vi "mode_sensitivity.vi"(0 "reference":refnum<class "OSA.lvclass">, 2 "sensitivity":T1=enum."high", 5 "error in (no error)":errorcluster, 9 "read/write":enum16{"read", "write"}(ring)) -> (14 "duplicate reference":refnum<class "OSA.lvclass">, 16 "sensitivity out":T1=enum."high", 19 "error out":errorcluster)   [LabVIEW 2010, in "OSA.lvclass"]
doc: "Sensitivity affect settable gain range, (sensitivity high: gain range = 0-15, and sens low: 0 - 11), and sampling intervall, (nr of samples per reference laser period, sens high: 32, low: 16). Sensitivity high recommended for low power sources or for high performance wavemeter resolution. The update rate, (interferogram read), is lower in high sensitivity mode."
uses:
  OSA.lvclass
  typeDef/sensitivityMode.ctl
  FTSLib.dll
panel:
  out "status":string
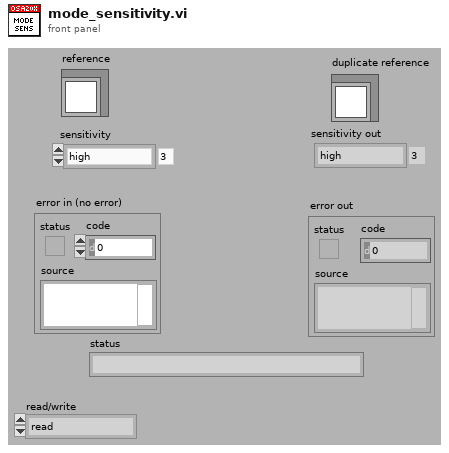
[diagram p1: front panel]
types:
  T1 = typedef "OSA.lvclass/sensitivityMode.ctl" = enum16{"low", "low medium", "high medium", "high"}
  T2 = typedef "OSA.lvclass/ObjectAttributes.ctl" = cluster{"Stop":bool, "dataType":T3, "spectrometerIdx":u16, "buffer size interferogram":i32, "interferogram":cluster{"new":bool, "plot_x_ min":sgl, "plot_x_max":sgl, "plot_y_min":sgl, "plot_y_max":sgl, "Graph Intrfrgrm":T4, "timeStamp":u32, "signal (%)":dbl, "traces":cluster{"idx":u32, "broadBand":bool, "monoChromatic":bool, "peakToPeakSignal":dbl, "peakToPeakPos":dbl}[], "traces idx last":i32}, "spectrum":cluster{"new":bool, "plot_x_min":sgl, "plot_x_max":sgl, "plot_unit_x":T5, "plot_unit_y":T6, "plot_y_min":sgl, "plot_y_max":sgl, "Graph Spectrum":T4, "timeStamp":u32, "X_VAL_OPTIONS":enum16{"MIN_MAX", "ARRAY"}, "traces":cluster{"idx":u32}[], "traces idx last":i32}, "Thorlabs_OSA_64.lvclass:queue_action.ctlqueue ref":refnum<queue>, "action":T7, "plot zoom step":dbl, "buffer semaphore":T8, "acq stopped":bool, "dataType active":T3, "temperature (degr C)":sgl, "pressure (hPa)":sgl, "rel humidity (%)":sgl, "settings":cluster{"resolution":T9, "sensitivity":T1, "Average":bool, "average nr":u32, "apodisation":T10, "acq delay (ms)":u32, "airMesure":T11, "wmtr on":bool, "intfgrm_smooth_width":u16, "intfgrm_smooth_nrOfPasses":u16, "intfgrm_smooth":T12, "phaseCorrection":T13, "zeroFill":u8, "spectr_smooth":T12, "spectr_smooth_width":u16, "spectr_smooth_nrOfPasses":u16, "resolution (/cm)":sgl, "REF wavelength, (nm)":dbl, "gain_idx":u16, "gainAuto":bool, "gain_relative":dbl, "PD sensitivity mode":T14, "PD senseMode implemented":bool, "SensorTemperature implemented":bool, "SensorPressure implemented":bool, "SensorHumidity implemented":bool}, "peaks position":sgl[], "peaks width":sgl[], "peaks height":sgl[], "peaks max nr":u32, "peaks latest nr":i32, "peaks new":bool, "power":dbl, "power new":bool, "path":string, "wavelength (WNr)":dbl, "wavelength new":bool, "buffer size spectrum":i32, "status":string, "VI reference":refnum<vi>, "funcPointer":u64, "libraryPointer":u64, "singleAcquisition":bool, "coherenceLength (cm)":dbl, "coherenceLength new":bool, "spectrometer model":string, "spectrometer serial nr":string, "peaks thld left":sgl[], "peaks thld right":sgl[], "coherenceLength error (cm)":dbl, "ADC bits":u16, "peaks position centroid":sgl[], "peaks height centroid":sgl[], "OSA series":T15, "channel":u16, "channels_nr":i32, "channel stiched":u32, "channelType_spectrum":T16}
  T3 = typedef "OSA.lvclass/acq_dataType.ctl" = enum16{"none", "interferogram", "spectrum"}
  T4 = typedef "OSA.lvclass/graph_intensity.ctl" = refnum<vi>
  T5 = typedef "OSA.lvclass/spectrum_x_unit.ctl" = enum16{"wavenr/cm", "THz", "eV", "nm_air", "nm_vac"}
  T6 = typedef "OSA.lvclass/y_unit.ctl" = enum16{"ADC counts", "dBm pwr absolute", "dBm pwr density", "mW pwr absolute", "mW pwr density"}
  T7 = typedef "OSA.lvclass/queue_action.ctl" = enum16{"none", "stop", "GUI_plotInterferogram", "GUI_plotSpectrum", "GUI_plotInterferogramRescale", "GUI_plotSpectrumRescale", "GUI_plotInterferogramReset", "GUI_plotSpectrumReset", "GUI_plotInterferogramAutoScaleY", "GUI_plotSpectrumAutoScaleY", "GUI_plotInterferogramZoomOut", "GUI_plotSpectrumZoomOut", "GUI_plotInterferogramPane", "GUI_plotSpectrumPane", "GUI_plotInterferogramZoomMouse", "GUI_plotSpectrumZoomMouse", "ENVIRONMENT temperature", "ENVIRONMENT pressure", "MODE_resolution set", "MODE_resolution get", "MODE_sensitivity set", "MODE_sensitivity get", "MODE_PDTemperature set", "MODE_PDTemperature get", "REBOOT/RESET firmware", "ACQASYNC_acquireSingleSpectrum", "ACQASYNC_continuous start", "ACQASYNC_continuous stop\n", "ACQASYNC_get last interferogram", "ACQASYNC_get last spectrum", "ACQASYNC_get last waveNr", "ACQOPT_interferogram smoothing set", "ACQOPT_interferogram smoothing get", "ACQOPT_spectrum smoothing set", "ACQOPT_spectrum smoothing get", "ACQOPT_apodisation type set", "ACQOPT_apodisation type get", "ACQOPT_phase correction type set", "ACQOPT_phase correction type get", "ACQOPT_acqIntervall_set", "ACQOPT_acqIntervall_get", "ACQOPT_average spectrum set", "ACQOPT_average spectrum get", "ACQOPT_rolling average set", "ACQOPT_rolling average get", "ACQOPT_zero fill factor set", "ACQOPT_zero fill factor get", "ACQOPT_cycle counting set", "ACQOPT_cycle counting get", "ACQOPT_air measure option set", "ACQOPT_air measure option get", "ACQOPT_gainLevel auto get", "ACQOPT_gainLevel auto set", "ACQOPT_gainLevel get", "ACQOPT_gainLevel set", "ACQOPT_getAll", "INSTRUMENT_PROPERTY_range_WaveNr_min", "INSTRUMENT_PROPERTY_range_WaveNr_max", "INSTRUMENT_PROPERTY_reference_wavelength_cm^-1", "INSTRUMENT_PROPERTY_samplesPerRefPeriod", "INSTRUMENT_PROPERTY_resolution_waveNrPercm", "INSTRUMENT_PROPERTY_availableGainLevels", "INSTRUMENT_PROPERTY_status", "CONVERT", "ANALYSE_POWER", "ANALYSE_PEAKS", "ANALYSE_WAVELENGTH", "ANALYSE_SPECTRUM", "ANALYSE_INTERFEROGRAM", "ANALYSE_COHERENCE_LENGTH", "MATH", "MATH_power", "MATH_peaks", "FILE", "miscellaneous"}
  T8 = typedef "Semaphore RefNum" = refnum<k1>
  T9 = typedef "OSA.lvclass/resolution.ctl" = enum16{"low", "high"}
  T10 = typedef "OSA.lvclass/apodisation.ctl" = enum16{"NONE", "NORTON_BEER_WEAK", "NORTON_BEER_MEDIUM", "NORTON_BEER_STRONG", "TRIANGULAR", "COSINE", "HANN", "HAMMING", "BLACKMANHARRIS3", "BLACKMANHARRIS4", "GAUSSIAN"}
  T11 = typedef "OSA.lvclass/airMeasure.ctl" = enum16{"TEMPERATURE", "PRESSURE"}
  T12 = typedef "OSA.lvclass/smoothing.ctl" = enum16{"NONE", "BINOMIAL", "SAVITSKY_GOLAY", "FOURIER", "MOVING_AVERAGE", "GAUSSIAN"}
  T13 = typedef "OSA.lvclass/phaseCorrection.ctl" = enum16{"NONE", "MERTZ", "FORMAN", "MERTZ_FILE", "FORMAN_FILE", "FUTURE COMP."}
  T14 = typedef "OSA.lvclass/PDTemperatureMode.ctl" = enum16{"cool: better sensitivity/noise floor", "warm: extended wl range"}
  T15 = typedef "OSA_series.ctl" = enum16{"OSA200", "OSA300", "UNKNOWN"}
  T16 = typedef "OSA.lvclass/channelType_spectrum.ctl" = enum16{"SINGLE CHANNEL", "STICHED"}
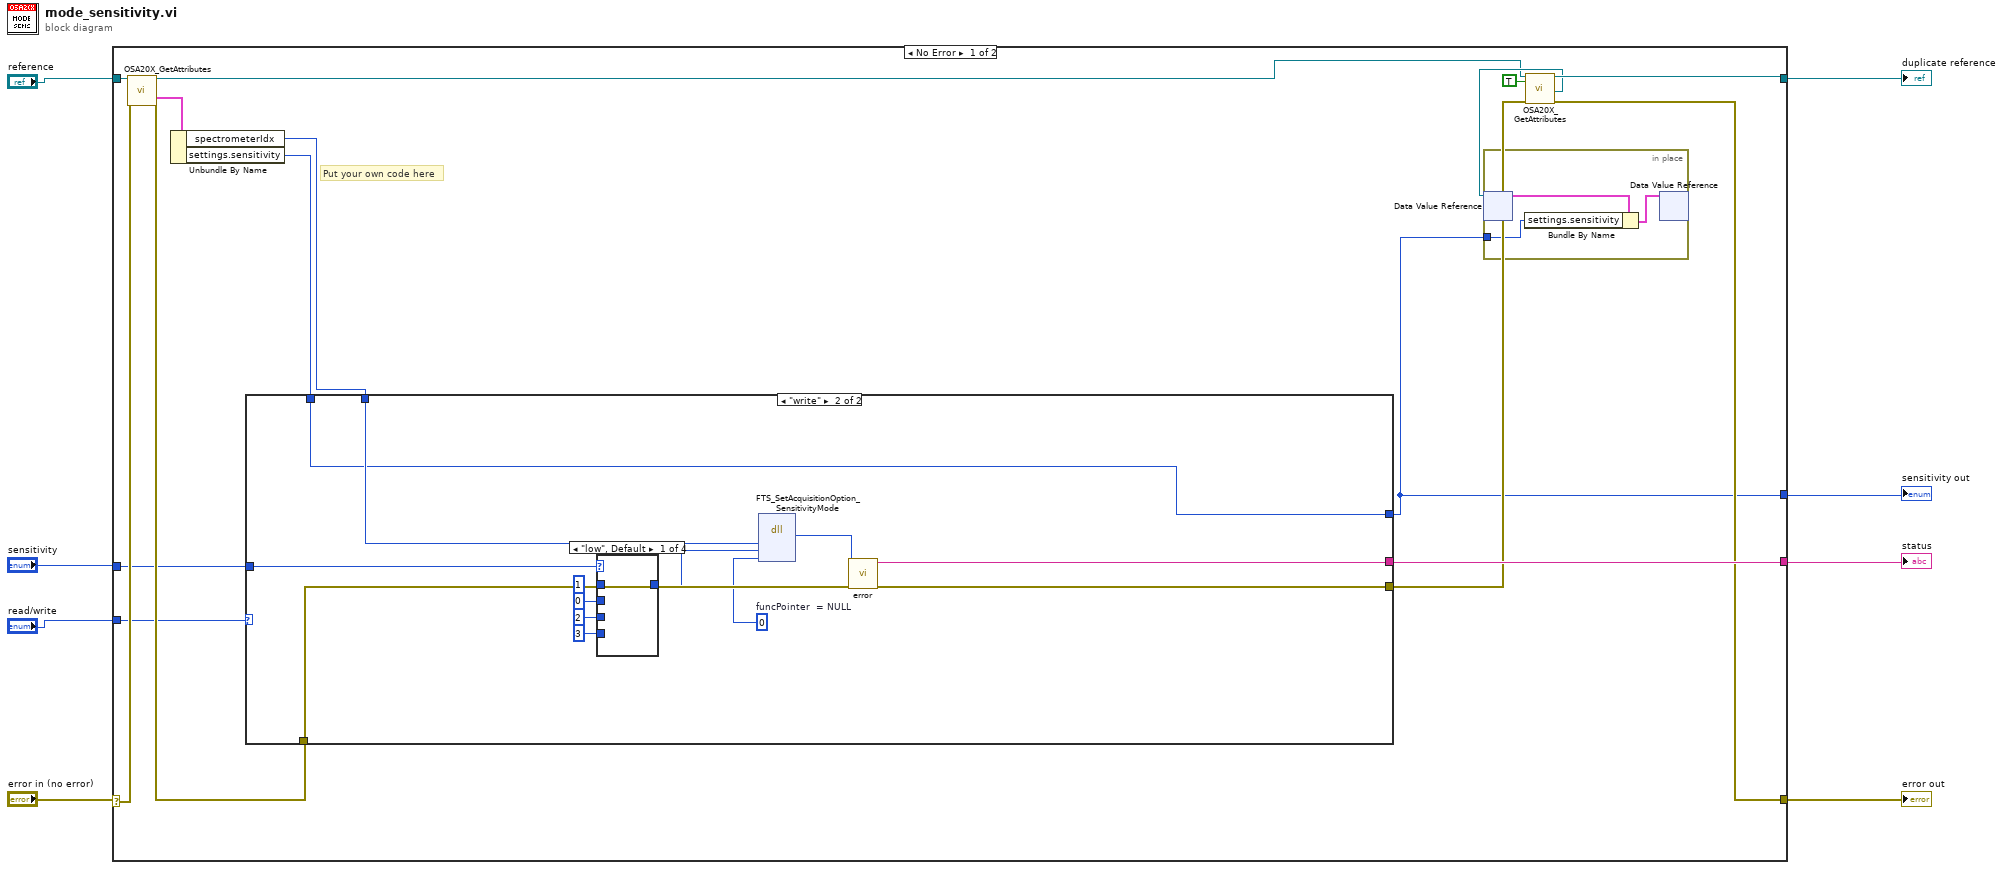
[diagram p0: block diagram]
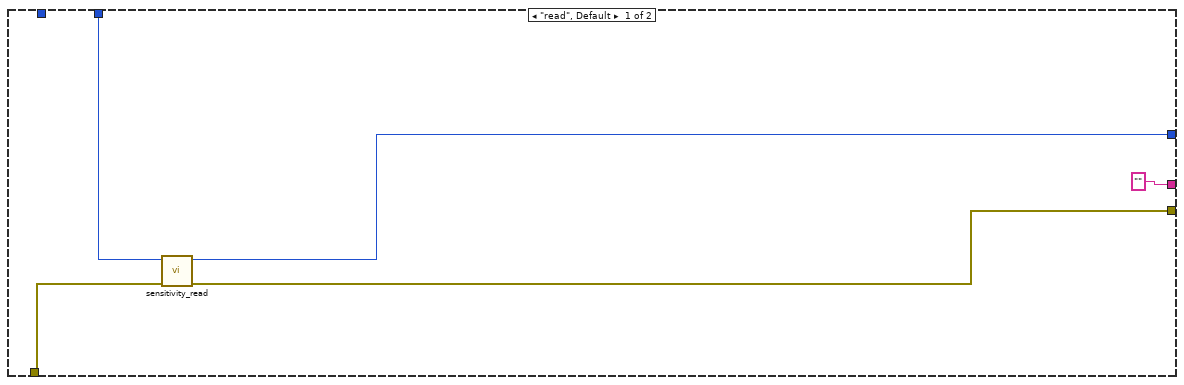
[diagram p2: hidden frame]
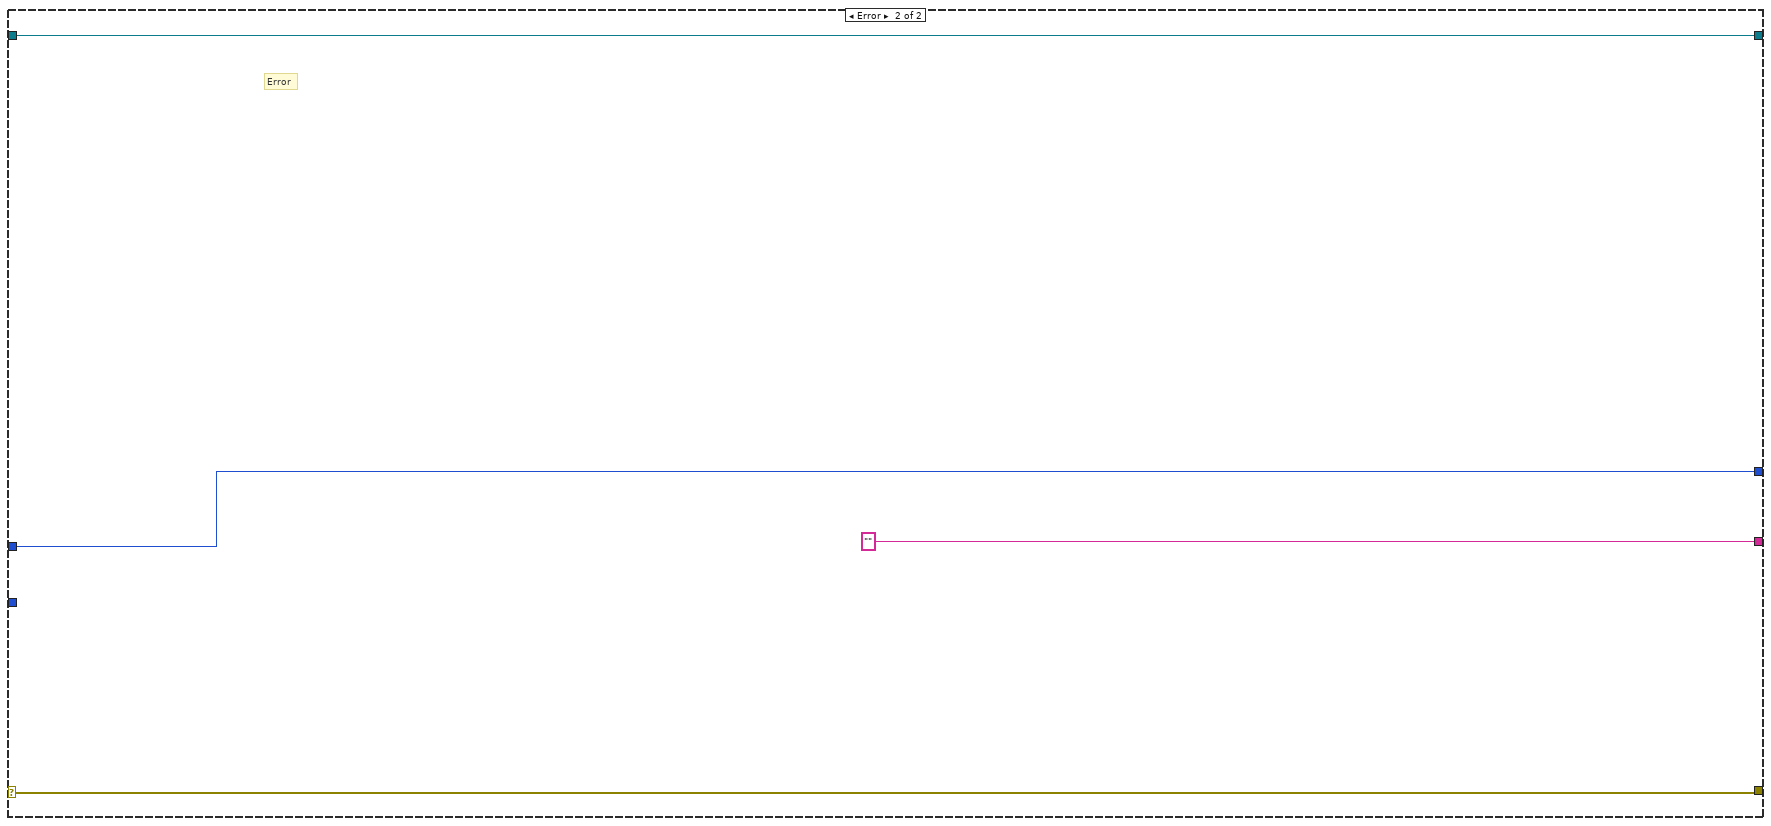
[diagram p6: hidden frame]
diagram:
  n1 = case shown="No Error" "error in (no error)" {
    selector: "error in (no error)" -> [w23 w52]
    tunnel: [w15 w52] -> w8
    tunnel: "reference" -> [w24 w53]
    tunnel: [w17 w53] -> w5
    tunnel: "sensitivity" -> [w18 w50]
    tunnel: [w21 "" ("status")] -> w3
    tunnel: "read/write" -> [w19 _]
    tunnel: [w10 w50] -> w1
    frame No Error {
      # "Put your own code here"
      n2 = call "OSA20X_GetAttributes.vi"("reference in"=w24, "error in (no error)"=w23) -> ("reference out"=w9:refnum<class "OSA.lvclass">, "Data"=w12:T2, "error out"=w22:errorcluster)  [unwired: 14 in, 1 out]
      n3 = Unbundle By Name(w12) -> ("spectrometerIdx"=w20:u16, "settings.sensitivity"=w14:T1)
      n4 = case shown="\"write\"" w19 {
        tunnel: w22 -> [w30 w44]
        tunnel: [w28 w35] -> w16
        tunnel: w18 -> [_ w37]
        tunnel: ["" ("status") w43] -> w21
        tunnel: w20 -> [w31 w42]
        tunnel: [w29 w34] -> w10
        tunnel: w14 -> [_ w34]
        frame "read", Default {
          n5 = call "sensitivity_read.vi"("error in (no error)"=w30, "spectrIdx"=w31) -> ("error out"=w28:errorcluster, "sensitivity"=w29:T1)  [unwired: 8 in]
        }
        frame "write" {
          w33 = u64 0  # funcPointer  = NULL
          n6 = case shown="\"low\", Default" w37 {
            tunnel: [w46 w47 w48 w49] -> w36
            tunnel: u16 1 -> [w46 _ _ _]
            tunnel: u16 0 -> [_ w47 _ _]
            tunnel: u16 2 -> [_ _ w48 _]
            tunnel: u16 3 -> [_ _ _ w49]
            frame "low", Default {
            }
            frame "low medium" {
            }
            frame "high medium" {
            }
            frame "high" {
            }
          }
          n7 = dll-call lib="FTSLib.dll" fn="FTS_SetAcquisitionOption_SensitivityMode"("spectrIdx"=w42, "sensitivityMode"=w36, "funcPointer"=w33) -> ("return type"=w45:i32)  [unwired: 6 in, 2 out]
          n8 = call "error.vi"("result code"=w45, "error in (no error)"=w44) -> ("status"=w43:string, "error out"=w35:errorcluster)  [unwired: 15 in, 1 out]
        }
      }
      n9 = call "OSA20X_GetAttributes.vi"("reference in"=w9, "OnlyGetDvrReference(False)"=TRUE, "error in (no error)"=w16) -> ("reference out"=w17:refnum<class "OSA.lvclass">, "DataRef"=w11:refnum<data-value>, "error out"=w15:errorcluster)  [unwired: 13 in, 1 out]
      n10 = in-place {
        in-place-border: w10 -> [w26]
        n11 = in-place-dvr #1(w11) -> (w27:T2)  [unwired: 1 out]
        n12 = Bundle By Name(cluster=w27, "settings.sensitivity"=w26) -> (w25:T2)
        n13 = in-place-dvr #1(w25) -> ()  [unwired: 2 out]
      }
    }
    frame Error {
      # "Error"
    }
  }
  "error out" <- w8
  "duplicate reference" <- w5
  "status" <- w3
  "sensitivity out" <- w1
